vi "On Target.vi"(11 "arm.lvclass":refnum<class "arm.lvclass">) -> (2 "On Target":bool, 3 "arm.lvclass":refnum<class "arm.lvclass">)   [LabVIEW 2015, in "arm.lvclass"]
uses:
  arm.lvclass
  arm.lvclass/arm.ctl
panel:
  in  "Angle":dbl=21.0 format="%#_13g"
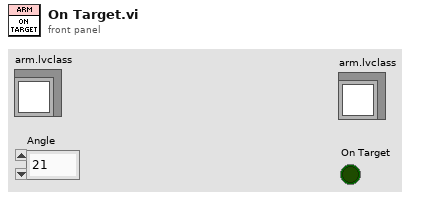
[diagram p1: front panel]
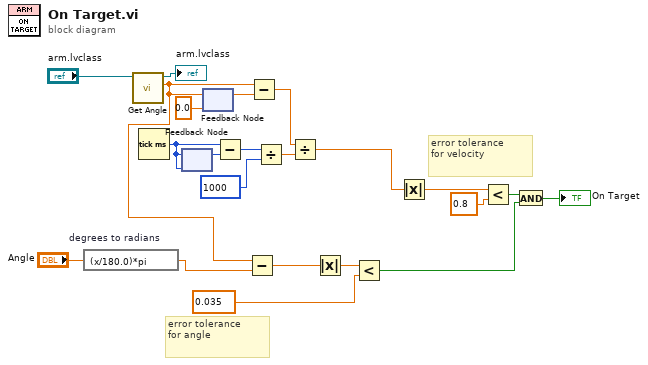
[diagram p0: block diagram]
diagram:
  # "error tolerance\nfor velocity"
  # "error tolerance\nfor angle"
  n1 = expression code="(x/180.0)*pi" "degrees to radians"("Angle") -> (w3:dbl)
  n2 = call "Get Angle.vi"("arm in"="arm.lvclass") -> ("Angle"=w2:dbl, "arm out"=→"arm.lvclass":refnum<class "arm.lvclass">)  [unwired: 9 in]
  n3 = Tick Count (ms)() -> (millisecond timer value=w16:u32)
  n4 = feedback #1(w16) -> (w15:u32)
  n5 = feedback-in #1(w16) -> ()
  n6 = feedback #2(0.0 ("Arm Angle")) -> (w19:dbl)
  n7 = feedback-in #2(w2) -> ()
  n8 = Subtract(x=w16, y=w15) -> (x-y=w17:u32)
  n9 = Subtract(x=w2, y=w3) -> (x-y=w7:dbl)
  n10 = Subtract(x=w2, y=w19) -> (x-y=w21:dbl)
  n11 = Divide(x=w17, y=u32 1000) -> (x/y=w22:dbl)
  n12 = Divide(x=w21, y=w22) -> (x/y=w14:dbl)
  n13 = Absolute Value(x=w7) -> (abs(x)=w6:dbl)
  n14 = Less?(x=w6, y=0.035) -> (x < y?=w9:bool)
  n15 = Absolute Value(x=w14) -> (abs(x)=w11:dbl)
  n16 = Less?(x=w11, y=0.8) -> (x < y?=w12:bool)
  n17 = And(x=w12, y=w9) -> (x .and. y?=→"On Target":bool)
